vi "mand iterator.vi"(10 "C":cdb, 11 "Number of iterations":dbl) -> (2 "Z out":i32)   [LabVIEW 2020]
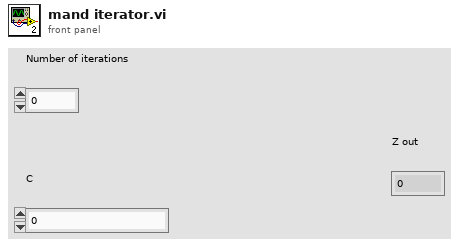
[diagram p1: front panel]
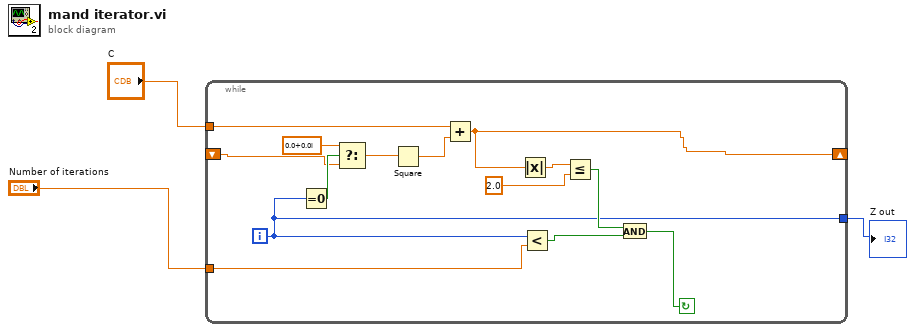
[diagram p0: block diagram]
diagram:
  n1 = while {
    shift-right: [w8] -> _
    shift-left: _ -> [w11]
    tunnel: "Number of iterations" -> [w14]
    tunnel: "C" -> [w13]
    tunnel: [w6] -> w1
    i -> [w6]
    stop <- w15 continue-if-true
    n2 = Equal To 0?(x=w6) -> (x = 0?=w12:bool)
    n3 = Select(t=cdb 0.0+0.0i, s=w12, f=w11) -> (s? t:f=w10:cdb)
    n4 = Square(x=w10) -> (x^2=w7:cdb)
    n5 = Add(x=w13, y=w7) -> (x+y=w8:cdb)
    n6 = Absolute Value(x=w8) -> (abs(x)=w4:dbl)
    n7 = Less?(x=w6, y=w14) -> (x < y?=w16:bool)
    n8 = Less Or Equal?(x=w4, y=2.0 ("x")) -> (x <= y?=w17:bool)
    n9 = And(x=w17, y=w16) -> (x .and. y?=w15:bool)
  }
  "Z out" <- w1
